vi "LoadConf.vi"(8 "error in":errorcluster, 10 "MEC":string, 11 "Device in":refnum<class "Device.lvclass">) -> (0 "error out":errorcluster, 3 "Device out":refnum<class "Device.lvclass">)   [LabVIEW 2012, in "Device.lvclass"]
uses:
  Device.lvclass
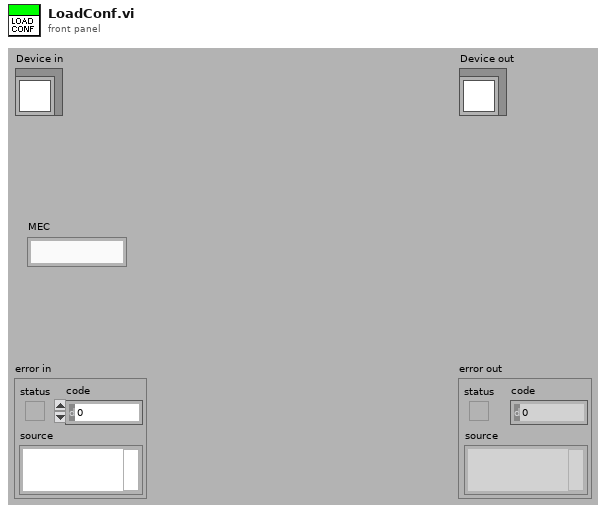
[diagram p1: front panel]
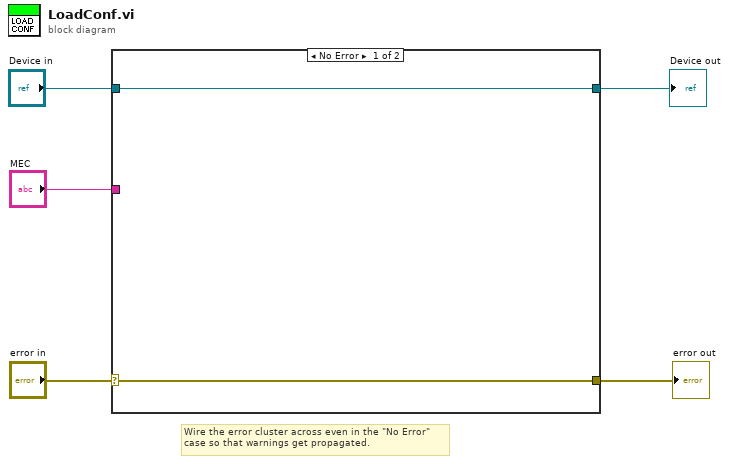
[diagram p0: block diagram]
diagram:
  # "Wire the error cluster across even in the \"No Error\"\ncase so that warnings get propagated."
  n1 = case shown="No Error" "error in" {
    selector: "error in" -> [w7 w9]
    tunnel: [w7 w9] -> w5
    tunnel: [w6 w8] -> w1
    tunnel: "MEC" -> [_ _]
    tunnel: "Device in" -> [w6 w8]
    frame No Error {
    }
    frame Error {
    }
  }
  "error out" <- w5
  "Device out" <- w1
